vi "Result.Test Result to SFC1.vi"(8 "error in":errorcluster, 9 "Test Result":T1={"#attributes"={"Version"="MTE_1.0.0"}, "Station"={"Name"="", "PN"="", "SN"="", "Rev"="", "PC Name"="", "Location"="", "HW_Config"={"HW_Item"=[]}, "SW_Config"={"SW_Item"=[]}}, "Test Run"={"Operator"="", "Start Time"=timestamp(0 s since 1904-01-01), "Duration(s)"=0.0, "Mode"="", "Comment"="", "ProcessStep"=""}, "Test Sequence"={"Name"="", "Config"={"Config_Item"=[]}}, "UUTs"={"UUT"=[]}} {"UUTs"."UUT"."Measurements"."Measurement"."Status" items=["LOG", "PASS", "FAIL", "ERROR"]}, 10 "File Name":string, 11 "Dir":path) -> (0 "error out":errorcluster, 3 "Report Path":path)   [LabVIEW 2018]
uses:
  Result XML/TestResult.FullResultData.ctl
  Result XML/TestResult.Station Info.ctl
  Result XML/TestResult.HW Item.ctl
  Result XML/TestResult.SW Item.ctl
  Result XML/TestResult.Test Run Info.ctl
  Result XML/TestResult.Test Info.ctl
  Result XML/TestResult.UUT Result.ctl
  Result XML/TestResult.Symptom.ctl
  Result XML/TestResult.Symptom.State.ctl
  Result.Measurement Item.ctl
  Result.Measurement and Attribute Item Status.ctl
  Result XML/TestResult.UUTInfo.ctl
  <vilib>/KATE/Files/File Utils.lvlib
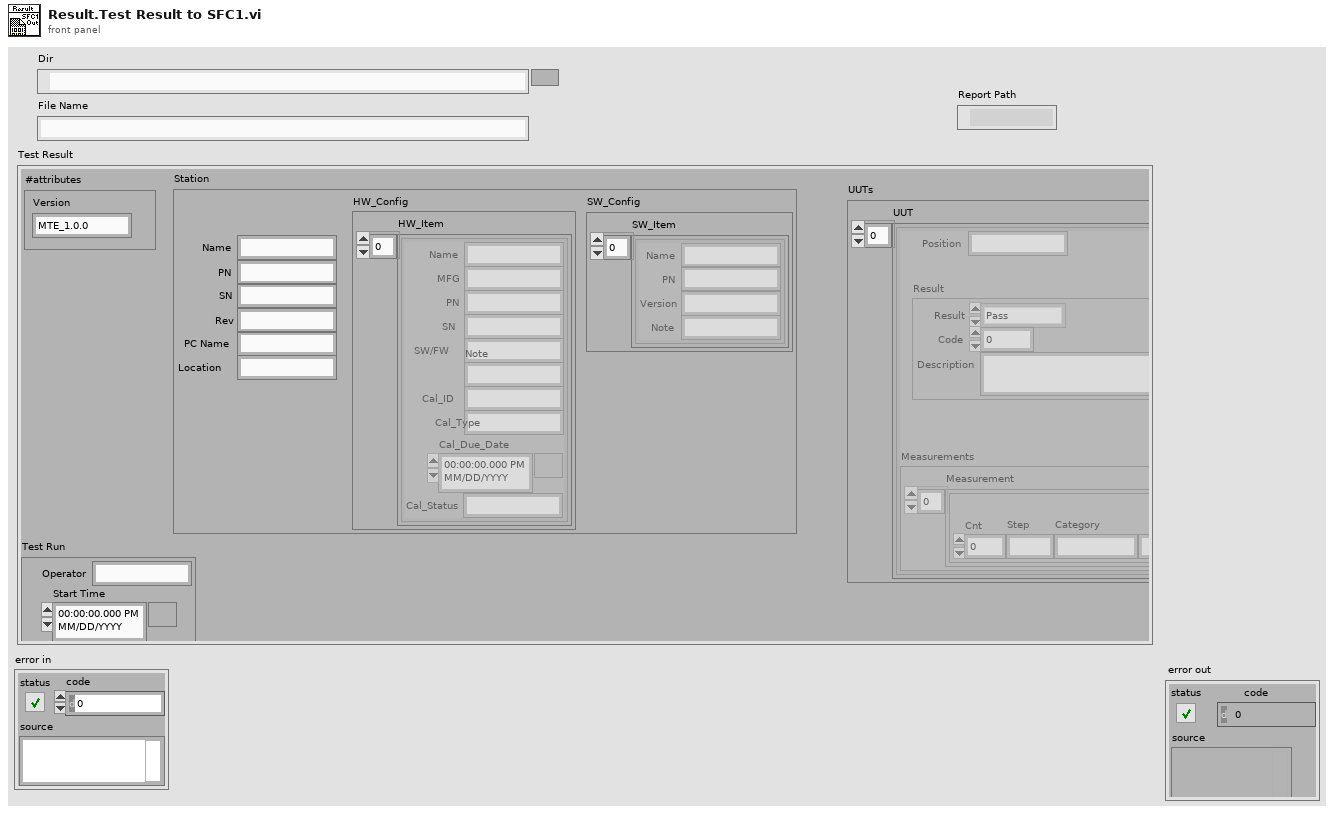
[diagram p1: front panel]
types:
  T1 = typedef "TestResult.FullResultData.ctl" = cluster{"#attributes":cluster{"Version":string}, "Station":T2, "Test Run":T5, "Test Sequence":T6, "UUTs":cluster{"UUT":T7[]}}
  T2 = typedef "TestResult.Station Info.ctl" = cluster{"Name":string, "PN":string, "SN":string, "Rev":string, "PC Name":string, "Location":string, "HW_Config":cluster{"HW_Item":T3[]}, "SW_Config":cluster{"SW_Item":T4[]}}
  T3 = typedef "TestResult.HW Item.ctl" = cluster{"Name":string, "MFG":string, "PN":string, "SN":string, "SW/FW":string, "Note":string, "Cal_ID":string, "Cal_Type":string, "Cal_Due_Date":timestamp, "Cal_Status":string}
  T4 = typedef "TestResult.SW Item.ctl" = cluster{"Name":string, "PN":string, "Version":string, "Note":string}
  T5 = typedef "TestResult.Test Run Info.ctl" = cluster{"Operator":string, "Start Time":timestamp, "Duration(s)":dbl, "Mode":string, "Comment":string, "ProcessStep":string}
  T6 = typedef "TestResult.Test Info.ctl" = cluster{"Name":string, "Config":cluster{"Config_Item":cluster{"Name":string, "Value":string}[]}}
  T7 = typedef "TestResult.UUT Result.ctl" = cluster{"Position":string, "Result":T8, "Measurements":cluster{"Measurement":T10[]}, "UUTInfo":T12}
  T8 = typedef "TestResult.Symptom.ctl" = cluster{"Result":T9, "Code":i32, "Description":string}
  T9 = typedef "TestResult.Symptom.State.ctl" = enum16{"Pass", "Fail", "Error", "Aborted", "Completed", "Logged"}
  T10 = typedef "Result.Measurement Item.ctl" = cluster{"Cnt":i32, "Step":string, "Category":string, "Name":string, "Value":string, "Units":string, "LimType":string, "LL":string, "UL":string, "Status":T11, "Code":i32, "Desc":string, "Time":timestamp}
  T11 = typedef "Result.Measurement and Attribute Item Status.ctl" = i32
  T12 = typedef "TestResult.UUTInfo.ctl" = cluster{"Product":string, "Desc":string, "PN":string, "SN":string, "Lot":string, "DateCode":string, "AltID":string, "Revision":string, "Properties":cluster{"Property":cluster{"Name":string, "Value":string}[]}}
  T13 = enum16{"open", "replace", "create", "open or create", "replace or create", "replace or create with confirmation"}
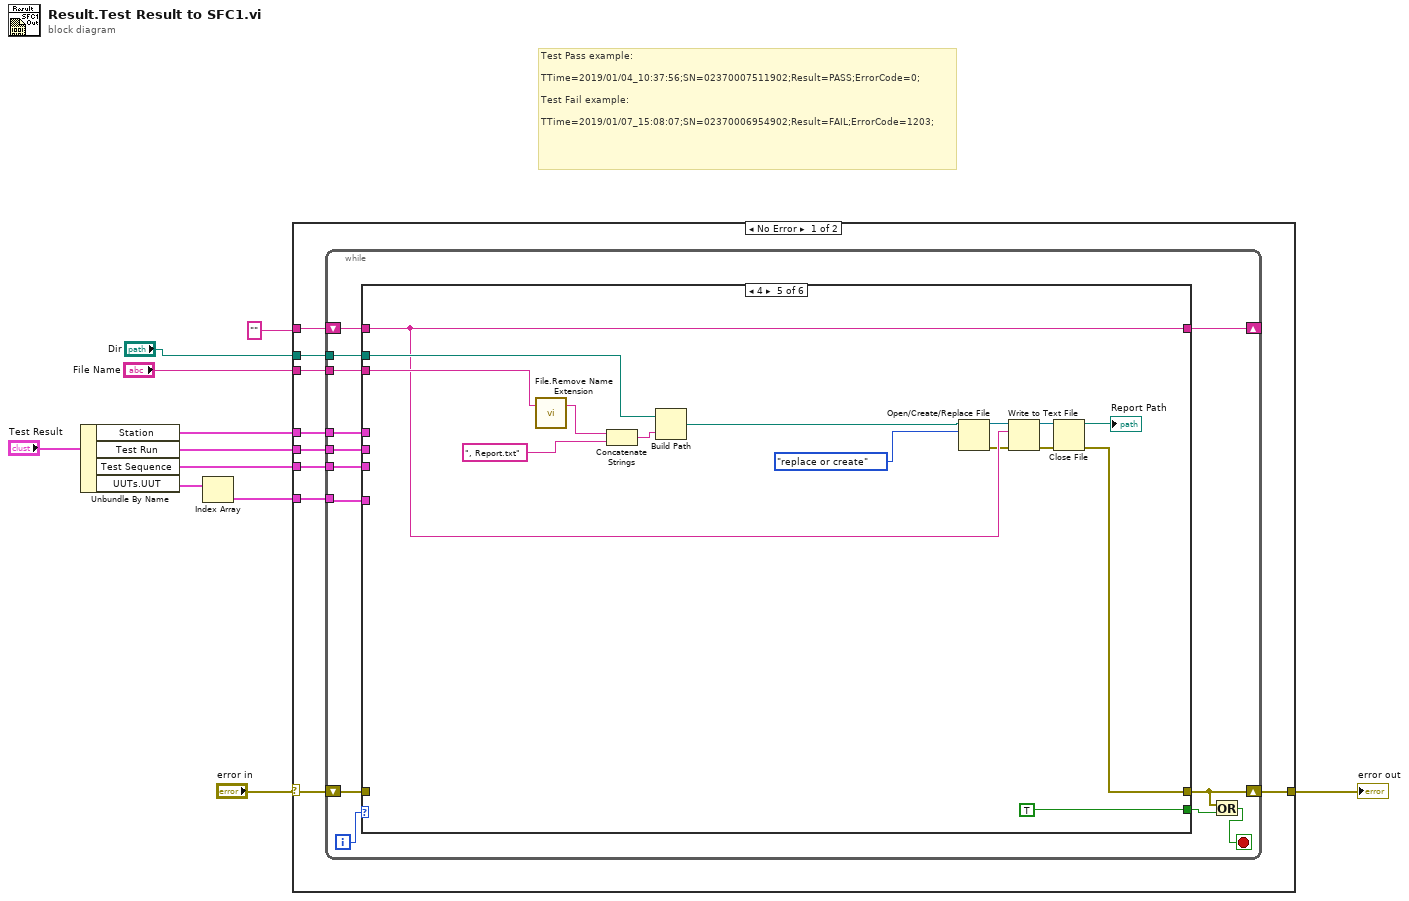
[diagram p0: block diagram]
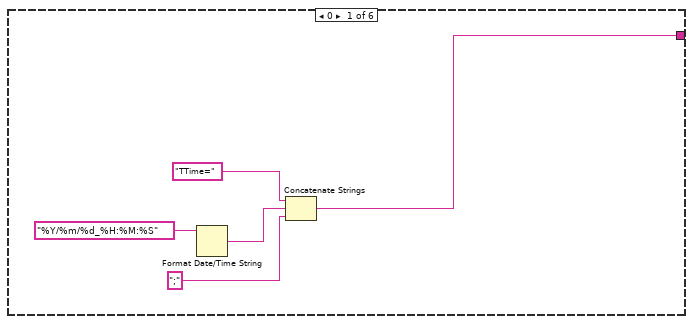
[diagram p2: hidden frame]
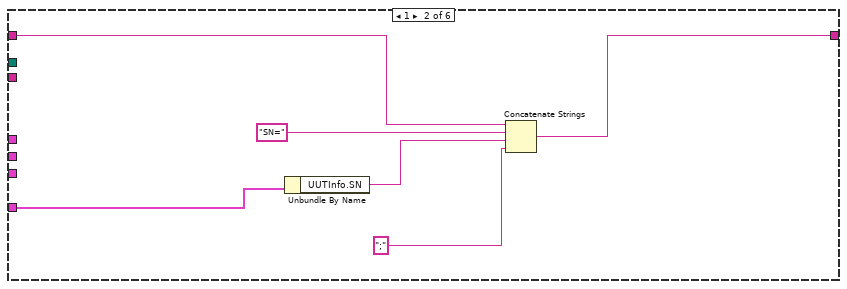
[diagram p3: hidden frame]
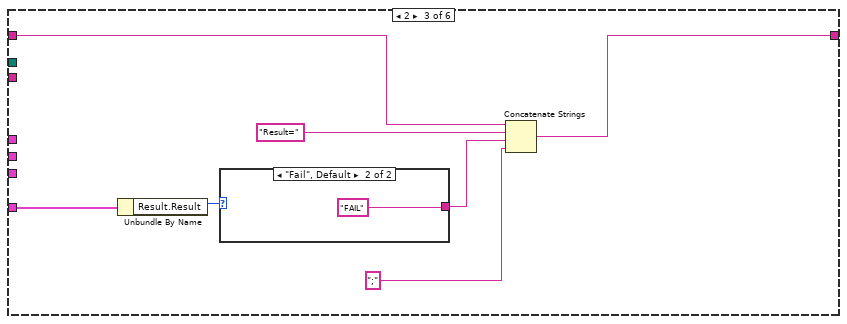
[diagram p4: hidden frame]
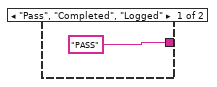
[diagram p5: hidden frame]
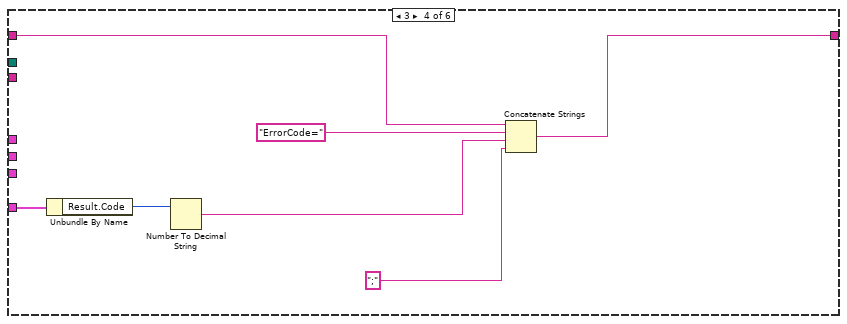
[diagram p6: hidden frame]
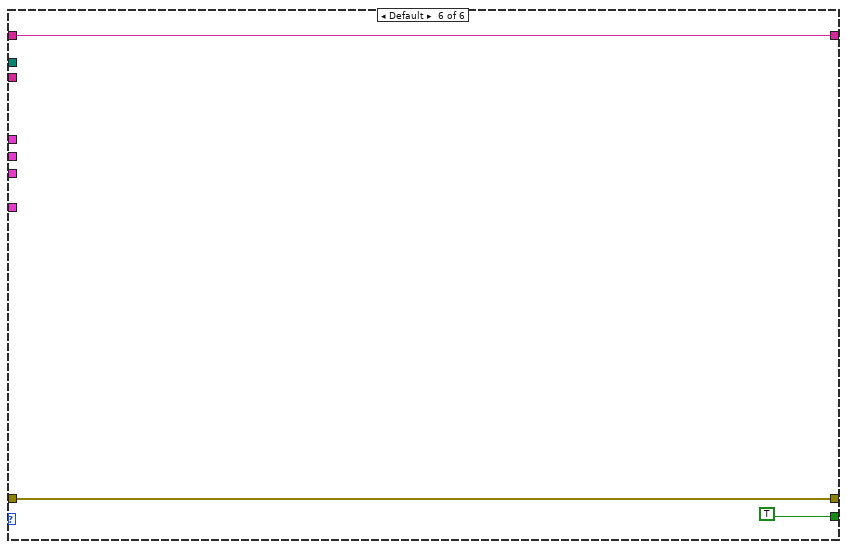
[diagram p7: hidden frame]
diagram:
  # "Test Pass example:\n\nTTime=2019/01/04_10:37:56;SN=02370007511902;Result=PASS;ErrorCode=0;\n\nTest Fail example:\n\nTTime=2019/01/07_15:08:07;SN=02370006954902;Result=FAIL;ErrorCode=1203;"
  n1 = Unbundle By Name("Test Result") -> ("Station"=w6:T2, "Test Run"=w5:T5, "Test Sequence"=w4:T6, "UUTs.UUT"=w8:T7[])
  n2 = Index Array(array=w8) -> (element=w7:T7)  [unwired: 1 in]
  n3 = case shown="No Error" "error in" {
    selector: "error in" -> [w19 w79]
    tunnel: [w20 w79] -> w11
    tunnel: w7 -> [w18 _]
    tunnel: w6 -> [w17 _]
    tunnel: w5 -> [w16 _]
    tunnel: w4 -> [w15 _]
    tunnel: "File Name" -> [w14 _]
    tunnel: "Dir" -> [w13 _]
    tunnel: "" -> [w12 _]
    frame No Error {
      n4 = while {
        shift-right: [w23] -> w20
        shift-left: w19 -> [w33]
        shift-right: [w26] -> _
        shift-left: w12 -> [w32]
        tunnel: w18 -> [w29]
        tunnel: w17 -> [w28]
        tunnel: w16 -> [w30]
        tunnel: w15 -> [w27]
        tunnel: w14 -> [w25]
        tunnel: w13 -> [w24]
        i -> [w31]
        stop <- w21 stop-if-true
        n5 = case shown="4" w31 {
          tunnel: [_ _ _ _ w69 w77] -> w23
          tunnel: w33 -> [_ _ _ _ _ w77]
          tunnel: w32 -> [_ w41 w48 w57 w66 w76]
          tunnel: [w34 w42 w49 w58 w66 w76] -> w26
          tunnel: w30 -> [_ _ _ _ _ _]
          tunnel: w29 -> [_ w40 w47 w56 _ _]
          tunnel: w28 -> [_ _ _ _ _ _]
          tunnel: w27 -> [_ _ _ _ _ _]
          tunnel: [_ _ _ _ TRUE TRUE] -> w22
          tunnel: w25 -> [_ _ _ _ w75 _]
          tunnel: w24 -> [_ _ _ _ w72 _]
          frame 0 {
            n6 = Format Date/Time String(time format string (%c)="%Y/%m/%d_%H:%M:%S") -> (date/time string=w36:string)  [unwired: 2 in]
            n7 = Concatenate Strings("TTime=", w36, ";") -> (w34:string)
          }
          frame 1 {
            n8 = Unbundle By Name(w40) -> ("UUTInfo.SN"=w39:string)
            n9 = Concatenate Strings(w41, "SN=", w39, ";") -> (w42:string)
          }
          frame 2 {
            n10 = Unbundle By Name(w47) -> ("Result.Result"=w46:T9)
            n11 = case shown="\"Fail\", Default" w46 {
              tunnel: ["PASS" "FAIL"] -> w45
              frame "Pass", "Completed", "Logged" {
              }
              frame "Fail", Default {
              }
            }
            n12 = Concatenate Strings(w48, "Result=", w45, ";") -> (w49:string)
          }
          frame 3 {
            n13 = Unbundle By Name(w56) -> ("Result.Code"=w55:i32)
            n14 = Number To Decimal String(number=w55) -> (decimal integer string=w54:string)  [unwired: 1 in]
            n15 = Concatenate Strings(w57, "ErrorCode=", w54, ";") -> (w58:string)
          }
          frame 4 {
            n16 = call <vilib>:"File.Remove Name Extension.vi"("File Name"=w75) -> ("Name Less Ext"=w68:string)  [unwired: 1 in, 1 out]
            n17 = Concatenate Strings(w68, ", Report.txt" ("string")) -> (w73:string)
            n18 = Build Path(base path=w72, name or relative path=w73) -> (appended path=w70:path)
            n19 = Open/Create/Replace File(file path (use dialog)=w70, operation (0:open)=T13."replace or create") -> (refnum out=w63:refnum<file>, error out=w64:errorcluster)  [unwired: 4 in, 1 out]
            n20 = Write to Text File(file (use dialog)=w63, text=w66, error in=w64) -> (refnum out=w62:refnum<file>, error out=w65:errorcluster)  [unwired: 1 in, 1 out]
            n21 = Close File(refnum=w62, error in=w65) -> (path=→"Report Path":path, error out=w69:errorcluster)
          }
          frame Default {
          }
        }
        n22 = Or(x=w23, y=w22) -> (x .or. y?=w21:bool)
      }
    }
    frame Error {
    }
  }
  "error out" <- w11
